vi "Controller.vi"(0 "y":dbl, 1 "Enable_Predicting_control":bool, 2 "CV":bool, 6 "SP":T3, 7 "real pwm rising edge":bool, 12 "model_v1_parameters":T2) -> (14 "CV":bool, 15 "error":bool, 16 "next state":T1, 17 "kLa out":dbl)   [LabVIEW 2021, in "MBPOnOff_Controller.lvlib"]
uses:
  MBPOnOff_Controller.lvlib
  typedefs/SetPoint.ctl
  Model_Predictor/typedefs/Model_v1_parameters.ctl
  typedefs/Controller_state.ctl
  Model_Predictor/Model_Predictor.lvclass
  Model_Predictor/typedefs/state_variables.ctl
  Model_Predictor/Model_Predictor.lvclass/Model_Predictor.ctl
  OUR_Monitor/OUR_Monitor.lvclass/OUR_Monitor.ctl
  Model_Predictor/Read So.vi
  Model_Predictor/Read kLa.vi
  Model_Predictor/Read Control_delay_buffer.vi
  Model_Predictor/Read dt.vi
  Model_Predictor/Read OUR.vi
  Model_Predictor/Read OUR_Monitor.vi
  OUR_Monitor/Read OUR.vi
  OUR_Monitor/Read OUR calculation threshold.vi
  Model_Predictor/Get Current_Acting_control.vi
  OUR_Monitor/OUR_Monitor.lvclass
panel:
  out "OUR calculation threshold":dbl
  out "OUR auto":dbl
  out "OUR":dbl
  in  "Update OUR":bool
  out "controls min":i16[](graph)
  out "controls max":i16[](graph)
  out "CONTROL_ON_due_to_prediction":bool
  out "CONTROL_OFF_due_to_prediction":bool
  out "size(s) 2":i32
  out "size(s)":i32
  out "index":i32
  out "calc_future_maximum":dbl[](graph)
  out "calc_future_minimum":dbl[](graph)
  out "state":T1
  out "Control_delay_buffer":bool[](array[boolean])
  out "So":dbl
  out "kLa":dbl
  out "Current_Acting_Control":bool
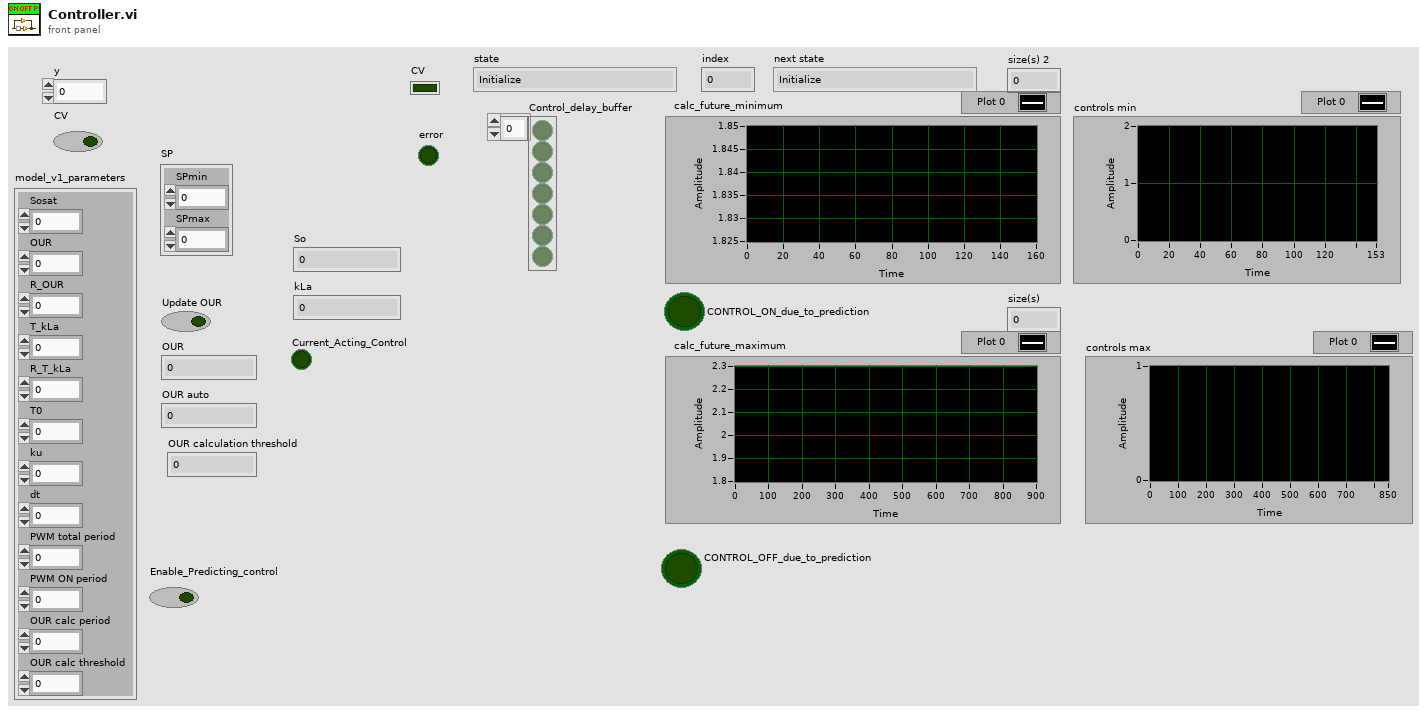
[diagram p1: front panel]
types:
  T1 = typedef "MBPOnOff_Controller.lvlib/Controller_state.ctl" = enum16{"Initialize", "Off_state", "Calculate_Future_Minimum", "On-State", "Calculate_Future_Maximum", "Error"}
  T2 = typedef "MBPOnOff_Controller.lvlib/Model_Predictor.lvclass/Model_v1_parameters.ctl" = cluster{"Sosat":dbl, "OUR":dbl, "R_OUR":dbl, "T_kLa":dbl, "R_T_kLa":dbl, "T0":dbl, "ku":dbl, "dt":dbl, "PWM total period":dbl, "PWM ON period":dbl, "OUR calc period":dbl, "OUR calc threshold":dbl}
  T3 = typedef "MBPOnOff_Controller.lvlib/SetPoint.ctl" = cluster{"SPmin":dbl, "SPmax":dbl}
  T4 = typedef "MBPOnOff_Controller.lvlib/Model_Predictor.lvclass/state_variables.ctl" = cluster{"So":dbl, "kLa":dbl}
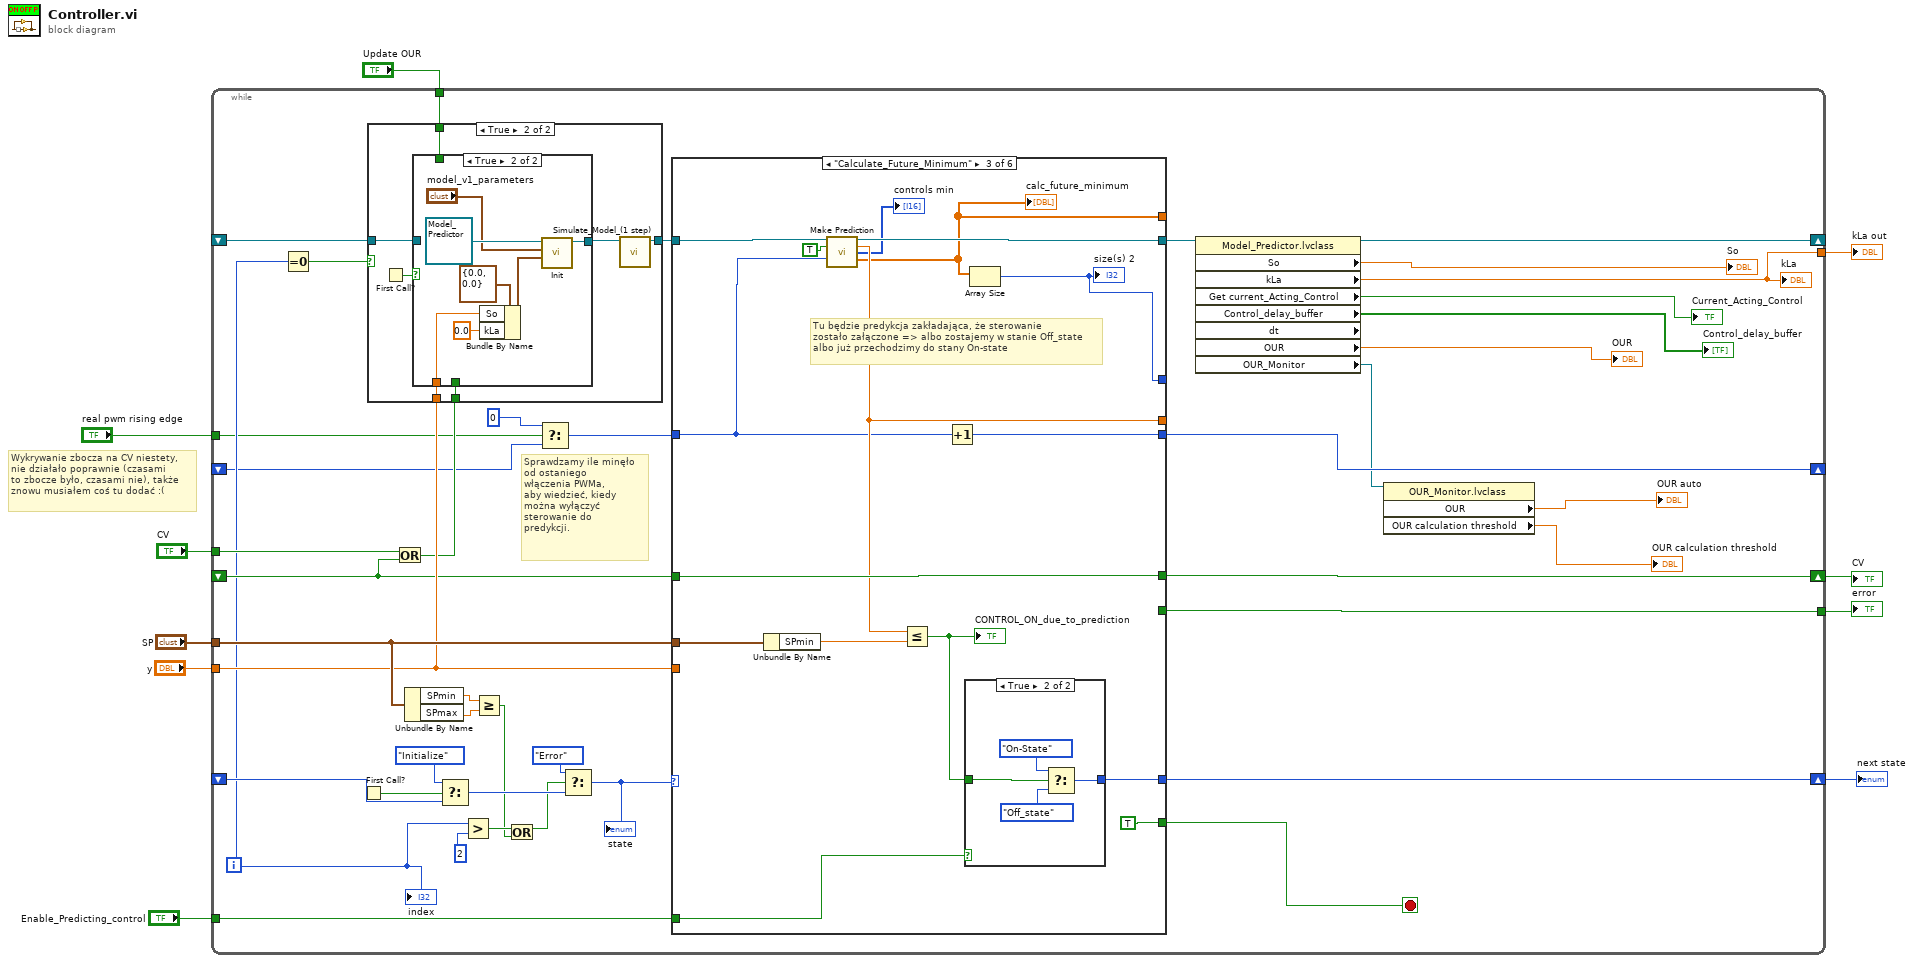
[diagram p0: block diagram]
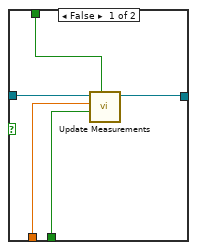
[diagram p3: hidden frame]
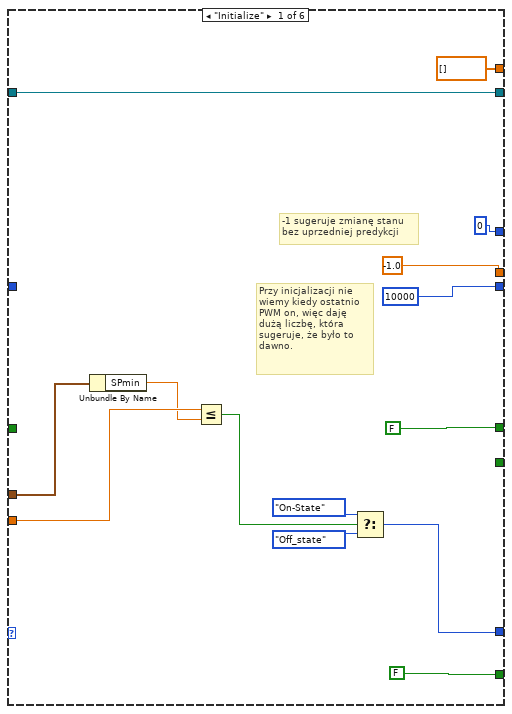
[diagram p4: hidden frame]
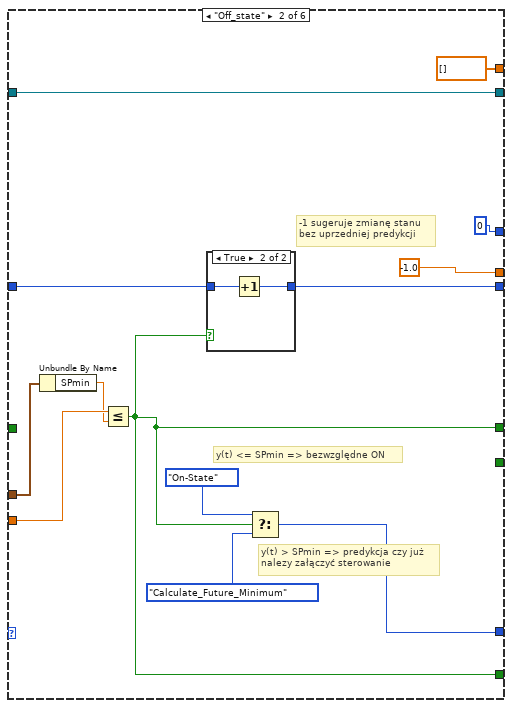
[diagram p5: hidden frame]
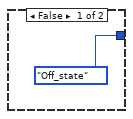
[diagram p7: hidden frame]
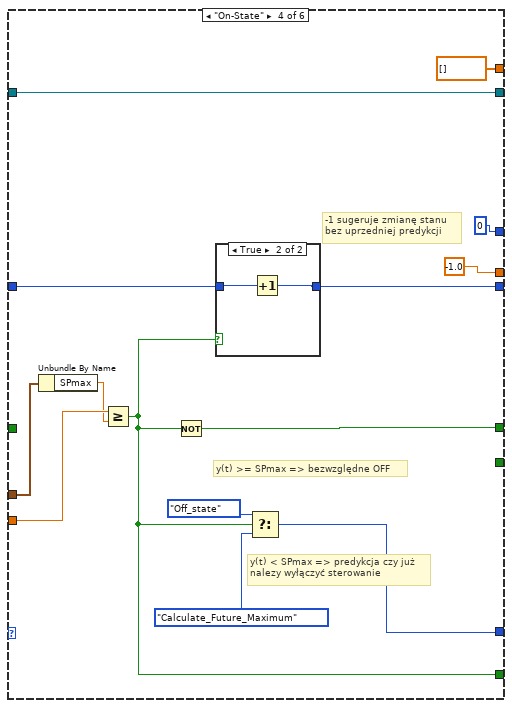
[diagram p8: hidden frame]
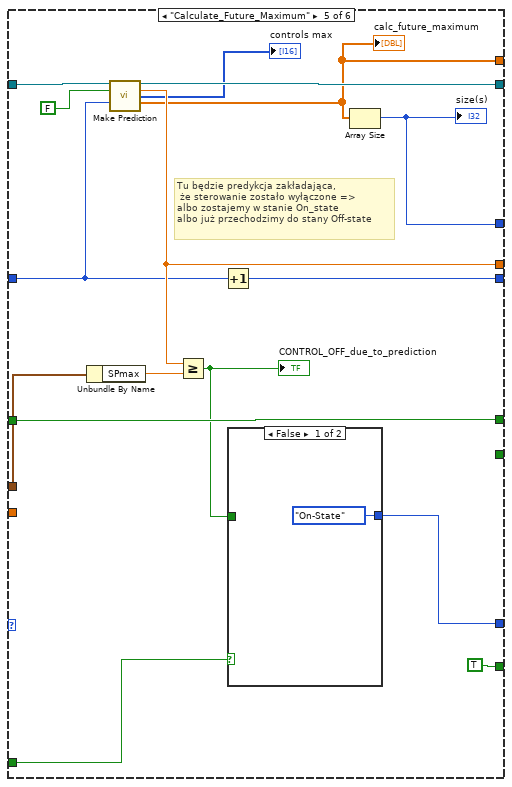
[diagram p10: hidden frame]
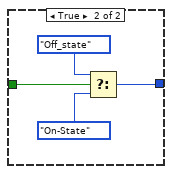
[diagram p11: hidden frame]
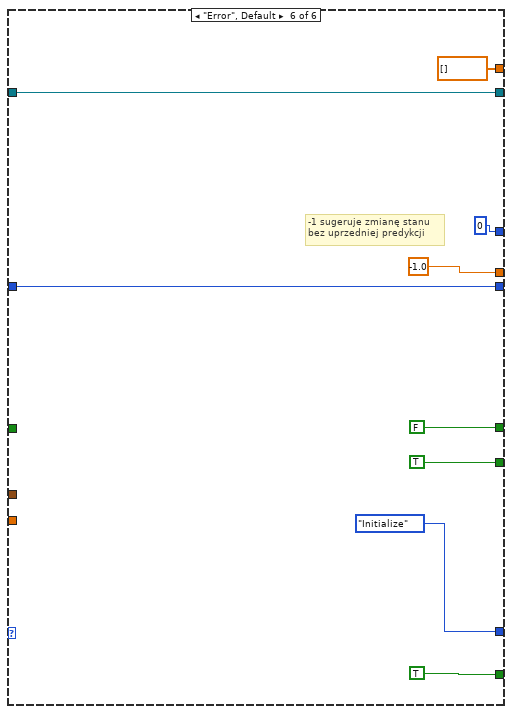
[diagram p12: hidden frame]
diagram:
  # "Wykrywanie zbocza na CV niestety,\nnie działało poprawnie (czasami\nto zbocze było, czasami nie), także\nznowu musiałem coś tu dodać :("
  n1 = while {
    shift-right: [w49] -> w4
    shift-left: _ -> [w51]
    tunnel: "y" -> [w35]
    tunnel: "SP" -> [w41]
    shift-right: [w17] -> w8
    shift-left: _ -> [w33]
    tunnel: [w42] -> w7
    shift-right: [w32] -> _
    shift-left: _ -> [w36]
    tunnel: "Enable_Predicting_control" -> [w27]
    tunnel: [w26] -> w5
    tunnel: "CV" -> [w24]
    shift-right: [w20] -> _
    shift-left: _ -> [w19]
    tunnel: "real pwm rising edge" -> [w18]
    tunnel: "Update OUR" -> [w16]
    i -> [w22]
    stop <- w50 stop-if-true
    # "Sprawdzamy ile minęło\nod ostaniego\nwłączenia PWMa,\naby wiedzieć, kiedy\nmożna wyłączyć\nsterowanie do\npredykcji."
    n2 = Equal To 0?(x=w22) -> (x = 0?=w28:bool)
    n3 = First Call?() -> (First Call?: T/F=w48:bool)
    n4 = Or(x=w24, y=w33) -> (x .or. y?=w25:bool)
    n5 = case shown="True" w28 {
      tunnel: w36 -> [w53 w59]
      tunnel: w35 -> [_ w58]
      tunnel: [w53 w56] -> w34
      tunnel: w25 -> [_ w55]
      tunnel: w16 -> [_ w54]
      frame False {
      }
      frame True {
        n6 = First Call?() -> (First Call?: T/F=w60:bool)
        n7 = case shown="True" w60 {
          tunnel: w59 -> [w65 _]
          tunnel: [w64 w71] -> w57
          tunnel: w58 -> [w63 w67]
          tunnel: w55 -> [w62 _]
          tunnel: w54 -> [w61 _]
          frame False {
            n8 = call "Update Measurements.vi"("Update OUR"=w61, "Control (aeration)"=w62, "So_measured"=w63, "Model_Predictor in"=w65) -> ("Model_Predictor out"=w64:refnum<class "Model_Predictor.lvclass">)  [unwired: 6 in, 1 out]
          }
          frame True {
            n9 = Bundle By Name(cluster=T4 {"So"=0.0, "kLa"=0.0} ("state_variables"), "So"=w67, "kLa"=0.0) -> (w68:T4)
            n10 = call "Init.vi"("state_variables"=w68, "model_v1_parameters"="model_v1_parameters", "Model_Predictor in"=refnum<class "Model_Predictor.lvclass"> refnum ("MBPOnOff_Controller.lvlib:Model_Predictor.lvclass")) -> ("Model_Predictor out"=w71:refnum<class "Model_Predictor.lvclass">)  [unwired: 7 in, 1 out]
          }
        }
        n11 = call "Simulate_Model_(1 step).vi"("Model_Predictor in"=w57) -> ("Model_Predictor out"=w56:refnum<class "Model_Predictor.lvclass">)  [unwired: 9 in, 1 out]
      }
    }
    n12 = Unbundle By Name(w41) -> ("SPmin"=w39:dbl, "SPmax"=w38:dbl)
    n13 = Select(t=Controller_state."Initialize" ("controller_state"), s=w48, f=w51) -> (s? t:f=w45:T1)
    n14 = Greater?(x=w22, y=2) -> (0:w46:bool)
    n15 = Greater Or Equal?(x=w39, y=w38) -> (x >= y?=w37:bool)
    n16 = Or(x=w46, y=w37) -> (x .or. y?=w40:bool)
    n17 = Select(t=0, s=w18, f=w19) -> (s? t:f=w23:i32)
    n18 = Select(t=Controller_state."Error", s=w40, f=w45) -> (s? t:f=w44:T1)
    "state" <- w44
    n19 = case shown="\"Calculate_Future_Minimum\"" w44 {
      tunnel: w35 -> [w85 w98 _ w136 _ _]
      tunnel: w41 -> [w86 w99 w115 w137 w151 _]
      tunnel: [w82 w95 w117 w133 w155 Controller_state."Initialize" ("f")] -> w49
      tunnel: [FALSE w90 TRUE w127 TRUE TRUE] -> w50
      tunnel: [FALSE w90 w111 w131 w149 FALSE] -> w17
      tunnel: w33 -> [_ _ w111 _ w149 _]
      tunnel: [_ _ _ _ _ TRUE] -> w42
      tunnel: w34 -> [w77 w93 w113 w130 w153 w166]
      tunnel: [w77 w93 w112 w130 w152 w166] -> w15
      tunnel: w27 -> [_ _ w110 _ w147 _]
      tunnel: [-1.0 -1.0 w108 -1.0 w146 -1.0] -> _
      tunnel: [10000 ("t") w88 w106 w125 w144 w164] -> w20
      tunnel: w23 -> [_ w89 w105 w126 w143 w164]
      tunnel: [0 0 w107 0 w145 0] -> _
      tunnel: [dbl[] [] ("Array") dbl[] [] ("Array") w103 dbl[] [] ("Array") w141 dbl[] [] ("Array")] -> _
      frame "Initialize" {
        # "Przy inicjalizacji nie wiemy kiedy ostatnio\nPWM on, więc daję dużą liczbę, która sugeruje, że było to dawno."
        # "-1 sugeruje zmianę stanu \nbez uprzedniej predykcji"
        n20 = Unbundle By Name(w86) -> ("SPmin"=w84:dbl)
        n21 = Less Or Equal?(x=w85, y=w84) -> (x <= y?=w83:bool)
        n22 = Select(t=Controller_state."On-State" ("controller_state"), s=w83, f=Controller_state."Off_state") -> (s? t:f=w82:T1)
      }
      frame "Off_state" {
        # "-1 sugeruje zmianę stanu \nbez uprzedniej predykcji"
        # "y(t) > SPmin => predykcja czy już\nnalezy załączyć sterowanie"
        # "y(t) <= SPmin => bezwzględne ON"
        n23 = Unbundle By Name(w99) -> ("SPmin"=w97:dbl)
        n24 = Less Or Equal?(x=w98, y=w97) -> (x <= y?=w90:bool)
        n25 = case shown="True" w90 {
          tunnel: w89 -> [w100 w102]
          tunnel: [w100 w101] -> w88
          frame False {
          }
          frame True {
            n26 = Increment(x=w102) -> (x+1=w101:i32)
          }
        }
        n27 = Select(t=Controller_state."On-State" ("controller_state"), s=w90, f=Controller_state."Calculate_Future_Minimum") -> (s? t:f=w95:T1)
      }
      frame "Calculate_Future_Minimum" {
        # "Tu będzie predykcja zakładająca, że sterowanie\nzostało załączone => albo zostajemy w stanie Off_state\nalbo już przechodzimy do stany On-state"
        n28 = Unbundle By Name(w115) -> ("SPmin"=w114:dbl)
        n29 = call "Make Prediction.vi"("Model_Predictor in"=w113, "Assumend_control"=TRUE, "Last PWM On"=w105) -> ("Model_Predictor out"=w112:refnum<class "Model_Predictor.lvclass">, "Achieved min or max"=w108:dbl, "Controls"=→"controls min":i16[], "Array"=w103:dbl[])  [unwired: 8 in, 1 out]
        "calc_future_minimum" <- w103
        n30 = Less Or Equal?(x=w108, y=w114) -> (x <= y?=w109:bool)
        "CONTROL_ON_due_to_prediction" <- w109
        n31 = Increment(x=w105) -> (x+1=w106:i32)
        n32 = case shown="True" w110 {
          tunnel: [Controller_state."Off_state" ("f") w121] -> w117
          tunnel: w109 -> [_ w120]
          frame False {
          }
          frame True {
            n33 = Select(t=Controller_state."On-State" ("controller_state"), s=w120, f=Controller_state."Off_state") -> (s? t:f=w121:T1)
          }
        }
        n34 = Array Size(array=w103) -> (size(s)=w107:i32)
        "size(s) 2" <- w107
      }
      frame "On-State" {
        # "-1 sugeruje zmianę stanu \nbez uprzedniej predykcji"
        # "y(t) < SPmax => predykcja czy już\nnalezy wyłączyć sterowanie"
        # "y(t) >= SPmax => bezwzględne OFF"
        n35 = Unbundle By Name(w137) -> ("SPmax"=w135:dbl)
        n36 = Greater Or Equal?(x=w136, y=w135) -> (x >= y?=w127:bool)
        n37 = Not(x=w127) -> (.not. x?=w131:bool)
        n38 = case shown="True" w127 {
          tunnel: w126 -> [w138 w140]
          tunnel: [w138 w139] -> w125
          frame False {
          }
          frame True {
            n39 = Increment(x=w140) -> (x+1=w139:i32)
          }
        }
        n40 = Select(t=Controller_state."Off_state" ("controller_state"), s=w127, f=Controller_state."Calculate_Future_Maximum") -> (s? t:f=w133:T1)
      }
      frame "Calculate_Future_Maximum" {
        # "Tu będzie predykcja zakładająca,\n że sterowanie zostało wyłączone => \nalbo zostajemy w stanie On_state\nalbo już przechodzimy do stany Off-state"
        n41 = Unbundle By Name(w151) -> ("SPmax"=w150:dbl)
        n42 = call "Make Prediction.vi"("Model_Predictor in"=w153, "Assumend_control"=FALSE, "Last PWM On"=w143) -> ("Model_Predictor out"=w152:refnum<class "Model_Predictor.lvclass">, "Achieved min or max"=w146:dbl, "Controls"=→"controls max":i16[], "Array"=w141:dbl[])  [unwired: 8 in, 1 out]
        "calc_future_maximum" <- w141
        n43 = Greater Or Equal?(x=w146, y=w150) -> (x >= y?=w148:bool)
        "CONTROL_OFF_due_to_prediction" <- w148
        n44 = Increment(x=w143) -> (x+1=w144:i32)
        n45 = case shown="False" w147 {
          tunnel: [Controller_state."On-State" ("f") w159] -> w155
          tunnel: w148 -> [_ w158]
          frame False {
          }
          frame True {
            n46 = Select(t=Controller_state."Off_state" ("controller_state"), s=w158, f=Controller_state."On-State") -> (s? t:f=w159:T1)
          }
        }
        n47 = Array Size(array=w141) -> (size(s)=w145:i32)
        "size(s)" <- w145
      }
      frame "Error", Default {
        # "-1 sugeruje zmianę stanu \nbez uprzedniej predykcji"
      }
    }
    n48 = property class="Model_Predictor.lvclass" props=["So", "kLa", "Get current_Acting_Control", "Control_delay_buffer", "dt", "OUR", "OUR_Monitor"](reference=w15) -> (reference out=w32:refnum<class "Model_Predictor.lvclass">, "So"=→"So":dbl, "kLa"=w26:dbl, "Get current_Acting_Control"=→"Current_Acting_Control":bool, "Control_delay_buffer"=→"Control_delay_buffer":bool[], "OUR"=→"OUR":dbl, "OUR_Monitor"=w13:refnum<class "OUR_Monitor.lvclass">)  [unwired: 1 in, 2 out]
    "kLa" <- w26
    n49 = property class="OUR_Monitor.lvclass"(reference=w13) -> ("OUR"=→"OUR auto":dbl, "OUR calculation threshold"=→"OUR calculation threshold":dbl)  [unwired: 1 in, 2 out]
    "index" <- w22
  }
  "CV" <- w8
  "error" <- w7
  "next state" <- w4
  "kLa out" <- w5
